vi "Pico Temperature.vi"() -> ()   [LabVIEW 2017]
panel:
  out "Temp 3":dbl
  out "Temp 2":dbl
  out "Temp 1":dbl
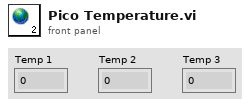
[diagram p1: front panel]
diagram:
